vi "Set Package BuildSpec Version.vi"(8 "error in (no error)":errorcluster, 9 "Build Specification Version":T1, 10 "package buildspec ref in":refnum<vi>, 11 "project ref in":refnum<vi>) -> (0 "error out":errorcluster, 1 "version updated?":bool, 2 "package buildspec ref out":refnum<vi>, 3 "project ref out":refnum<vi>)   [LabVIEW 2018, in "NIPKG BuildSpec API.lvlib"]
doc: "This VI sets the version of the specified dependency package in the Package build specification of a LabVIEW project.\n\nNote: To persist the updated version in the LabVIEW project file, you must Save the project after this VI finishes executing."
uses:
  NIPKG BuildSpec API.lvlib
  <vilib>/AppBuilder/AB_API_Simple/Build Specification Version.ctl
  <vilib>/AppBuilder/AB_API_Simple/NI_App_Builder_API.lvlib
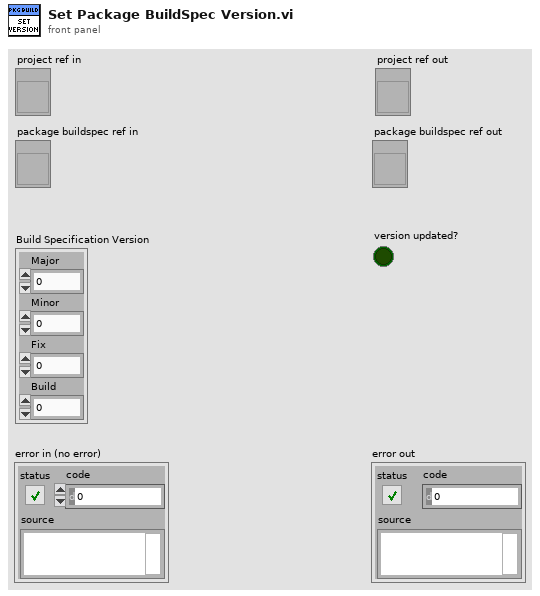
[diagram p1: front panel]
types:
  T1 = typedef "NI_App_Builder_API.lvlib/Build Specification Version.ctl" = cluster{"Major":u16, "Minor":u16, "Fix":u16, "Build":u16}
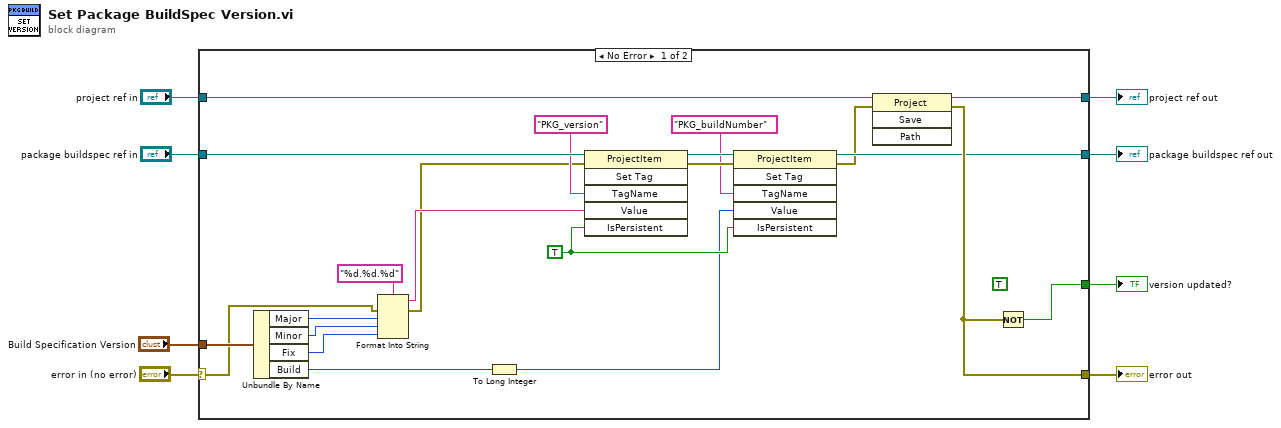
[diagram p0: block diagram]
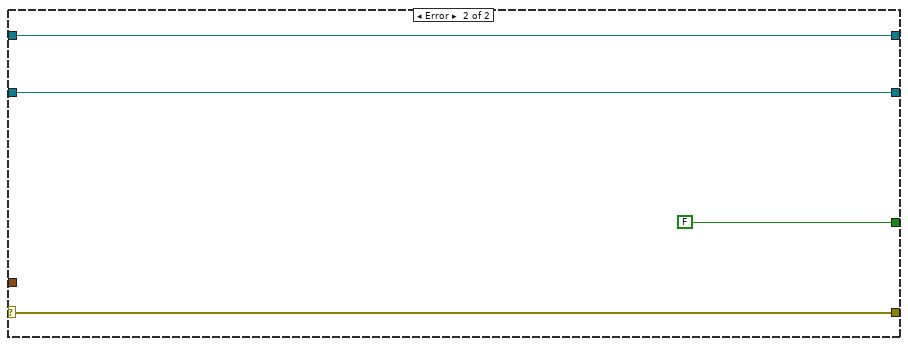
[diagram p2: hidden frame]
diagram:
  n1 = case shown="No Error" "error in (no error)" {
    selector: "error in (no error)" -> [w15 w34]
    tunnel: "package buildspec ref in" -> [w30 w31]
    tunnel: "Build Specification Version" -> [w27 _]
    tunnel: [w26 w34] -> w6
    tunnel: [w12 w31] -> w5
    tunnel: [w25 FALSE] -> w4
    tunnel: "project ref in" -> [w29 w32]
    tunnel: [w28 w32] -> w2
    frame No Error {
      (unwired) TRUE
      w16 = TRUE ("Is Persistent")
      n2 = Unbundle By Name(w27) -> ("Major"=w20:u16, "Minor"=w19:u16, "Fix"=w18:u16, "Build"=w10:u16)
      n3 = Format Into String(format string="%d.%d.%d", error in=w15, w20, w19, w18) -> (resulting string=w14:string, error out=w13:errorcluster)  [unwired: 1 in]
      n4 = To Long Integer(number=w10) -> (32bit integer=w9:i32)
      n5 = invoke class="ProjectItem" method="Set Tag"(reference=w30, error in=w13, "TagName"="PKG_version" ("format string"), "Value"=w14, "IsPersistent"=w16) -> (reference out=w23:refnum<vi>, error out=w24:errorcluster)  [unwired: 1 in, 4 out]
      n6 = invoke class="ProjectItem" method="Set Tag"(reference=w23, error in=w24, "TagName"="PKG_buildNumber" ("format string"), "Value"=w9, "IsPersistent"=w16) -> (reference out=w12:refnum<vi>, error out=w11:errorcluster)  [unwired: 1 in, 4 out]
      n7 = invoke class="Project" method="Save"(reference=w29, error in=w11) -> (reference out=w28:refnum<vi>, error out=w26:errorcluster)  [unwired: 2 in, 2 out]
      n8 = Not(x=w26) -> (.not. x?=w25:bool)
    }
    frame Error {
    }
  }
  "error out" <- w6
  "package buildspec ref out" <- w5
  "version updated?" <- w4
  "project ref out" <- w2
